vi "DetectorGlobals.vi"() -> ()   [LabVIEW 2014]
panel:
  out "NumFT":i32=1
  out "DarkRows":i32=1
  out "DarkCols":i32=1
  out "DevRows":i32=1
  out "DevCols":i32=1
  out "AmpConfig":string
  out "NDetY":i32
  out "NDetX":i32
  out "Splits":i32
  out "SetTemperature":dbl
  out "OverRows":i32
  out "UnderRows":i32
  out "OverCols":i32=20
  out "UnderCols":i32
  out "LastRow":i32=4064
  out "FirstRow":i32=1
  out "LastCol":i32=4064
  out "FirstCol":i32=1
  out "ColBin":i32=1
  out "RowBin":i32=1
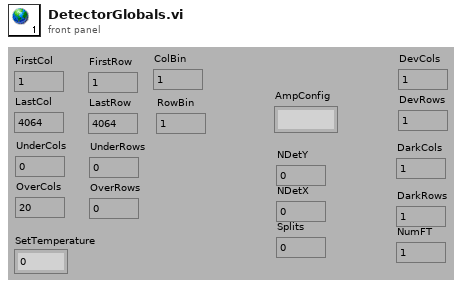
[diagram p1: front panel]
diagram:
